vi "FreeGPUandSLM.vi"(1 "error in":errorcluster) -> (0 "error out":errorcluster)   [LabVIEW 2009]
uses:
  GenerateHologramCUDA.dll
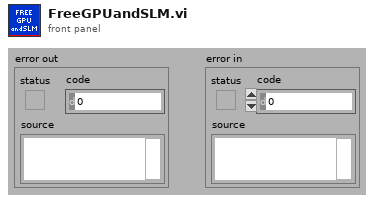
[diagram p1: front panel]
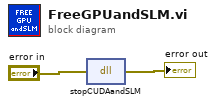
[diagram p0: block diagram]
diagram:
  n1 = dll-call lib="C:/Users/Martin/GenerateHologramCUDA/LabVIEW/GenerateHologramCUDA.dll" fn="stopCUDAandSLM"(error in="error in") -> (error out=→"error out":errorcluster)  [unwired: 2 in, 2 out]
